vi "数值循环.vi"(8 "加/减":bool, 9 "下限":dbl, 10 "上限":dbl, 11 "输入":dbl) -> (3 "输出":dbl)   [LabVIEW 2012]
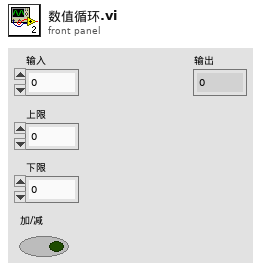
[diagram p1: front panel]
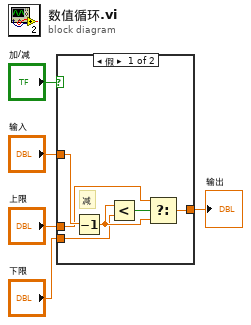
[diagram p0: block diagram]
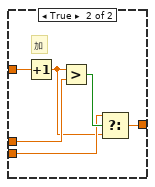
[diagram p2: hidden frame]
diagram:
  n1 = case shown="假" "加/减" {
    tunnel: "输入" -> [w9 w17]
    tunnel: "上限" -> [w7 w16]
    tunnel: "下限" -> [w8 w14]
    tunnel: [w6 w12] -> w1
    frame False {
      # "减"
      n2 = Decrement(x=w9) -> (x-1=w10:dbl)
      n3 = Less?(x=w10, y=w8) -> (x < y?=w11:bool)
      n4 = Select(t=w7, s=w11, f=w10) -> (s? t:f=w6:dbl)
    }
    frame True {
      # "加"
      n5 = Increment(x=w17) -> (x+1=w13:dbl)
      n6 = Greater?(x=w13, y=w16) -> (0:w15:bool)
      n7 = Select(t=w14, s=w15, f=w13) -> (s? t:f=w12:dbl)
    }
  }
  "输出" <- w1
